vi "总磷总氮启动参数对话框.vi"() -> (2 "确认":bool, 3 "元素":cluster{"命令":string, "data":variant})   [LabVIEW 2016, in "斯坦道总磷总氮.lvlib"]
uses:
  <vilib>/Utility/miscctls.llb/LVStringsAndValuesArrayTypeDef_U16.ctl
panel:
  out "标液值":dbl caption="标液值："
  in  "取消":bool
  in  "确定":bool
  in  "测量间隔":u16
  in  "模式设置":T1(ring)
  in  "量程切换":u16(ring)=2 items=["H", "L", "AUTO"]
  in  "站号":u16(ring)=1 items=["氨氮"=3, "总磷"=1]
  in  "控制命令":T2(ring)
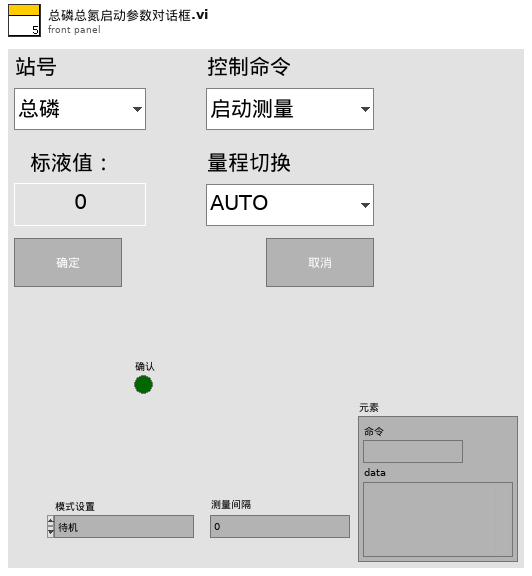
[diagram p1: front panel]
types:
  T1 = enum16{"待机", "连续模式", "周期模式", "定点模式", "受控模式", "手动模式"}
  T2 = enum16{"启动测量", "标样核查", "零点核查", "跨度核查", "空白测试", "平行样测试", "加标回收", "空白校准", "标样校准", "初始化（清洗）", "停止测试", "仪器重启", "校时", "模式设置", "测量间隔设置"}
  T3 = typedef "LVStringsAndValuesArrayTypeDef_U16.ctl" = cluster{"String":string, "Value":u16}[]
  T4 = cluster{"COD":bool, "氨氮":bool, "总氮":bool, "总磷":bool}
  T5 = cluster{"站号":u16, "量程切换":enum32{"H", "L", "AUTO"}, "控制命令":enum16{"启动测量", "标样核查", "零点核查", "跨度核查", "空白测试", "平行样测试", "加标回收", "空白校准", "标样校准", "初始化（清洗）", "停止测试", "仪器重启", "校时", "模式设置", "测量间隔设置", "盲样测试"}, "模式设置":enum16{"待机", "连续模式", "周期模式", "定点模式", "受控模式", "手动模式"}, "测量间隔":u16}
  T6 = cluster{"总磷跨度值":dbl, "总磷零点标准液浓度":dbl, "总磷跨度标准液浓度":dbl, "总磷标准液标准浓度":dbl, "总氮跨度值":dbl, "总氮零点标准液浓度":dbl, "总氮跨度标准液浓度":dbl, "总氮标准液标准浓度":dbl, "COD跨度值":dbl, "COD零点标准液浓度":dbl, "COD跨度标准液浓度":dbl, "COD标准液标准浓度":dbl, "氨氮跨度值":dbl, "氨氮零点标准液浓度":dbl, "氨氮跨度标准液浓度":dbl, "氨氮标准液标准浓度":dbl}
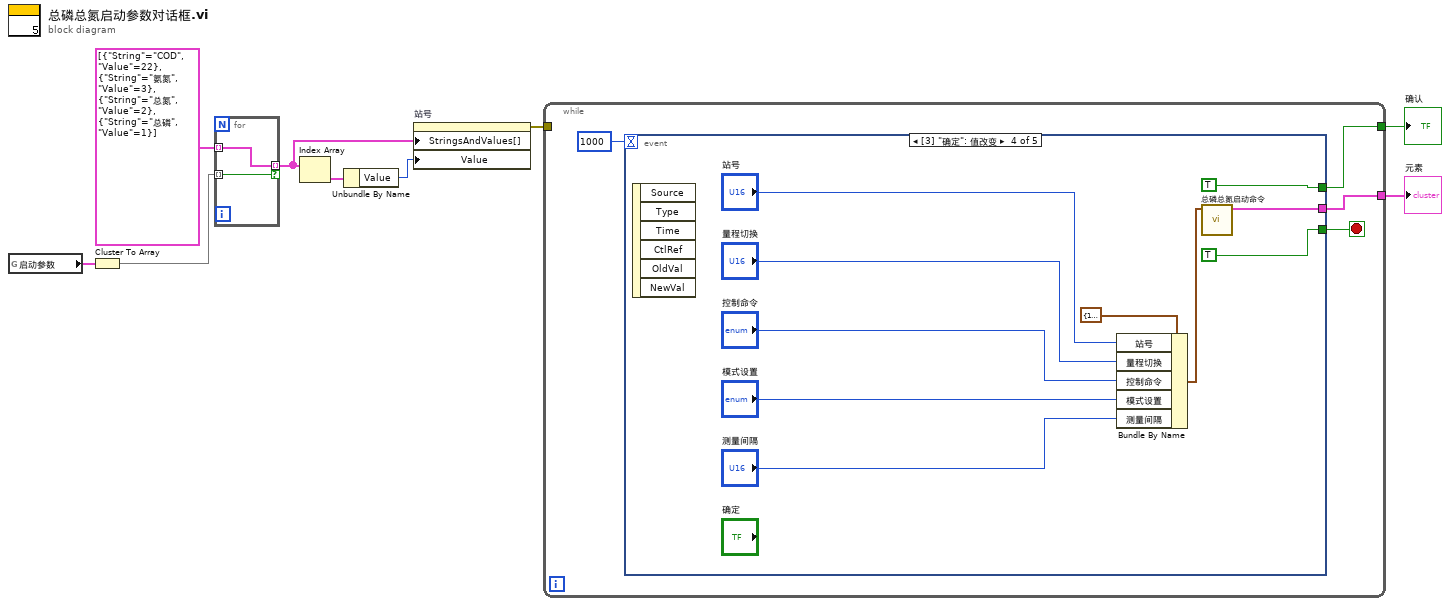
[diagram p0: block diagram]
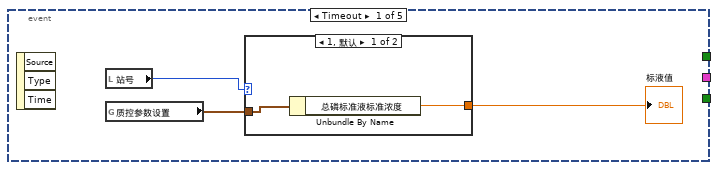
[diagram p2: hidden frame]
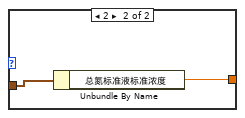
[diagram p3: hidden frame]
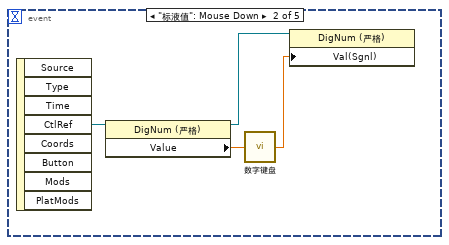
[diagram p4: hidden frame]
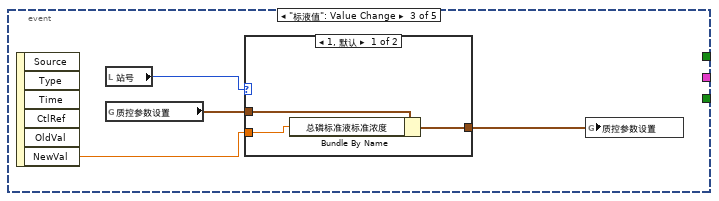
[diagram p5: hidden frame]
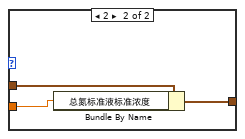
[diagram p6: hidden frame]
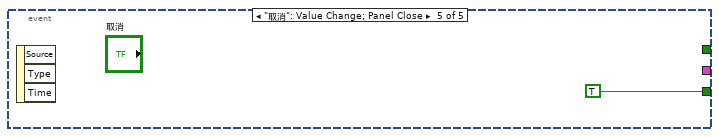
[diagram p7: hidden frame]
diagram:
  n1 = global read "总磷总氮断电保存全局变量.vi" "启动参数"() -> (w4:T4)
  n2 = Cluster To Array(cluster=w4) -> (array=w3:bool[])
  n3 = for {
    tunnel: w3 -> [w10] mode=indexing
    tunnel: T3 [{"String"="COD", "Value"=22}, {"String"="氨氮", "Value"=3}, {"String"="总氮", "Value"=2}, {"String"="总磷", "Value"=1}] ("字符串与值[]") -> [w11] mode=indexing
    tunnel: [w11] -> w1 mode=indexing if=w10
  }
  n4 = Index Array(array=w1) -> (element=w7:cluster{"String":string, "Value":u16})  [unwired: 1 in]
  n5 = Unbundle By Name(w7) -> ("Value"=w6:u16)
  n6 = property on="站号" class="Ring (严格)"("StringsAndValues[]"=w1, "Value"=w6) -> (error out=w5:errorcluster)  [unwired: 2 in, 1 out]
  n7 = while {
    tunnel: [w13] -> w9
    tunnel: [w12] -> w8
    tunnel: w5 -> [_]
    stop <- w15 stop-if-true
    n8 = event shown="[3] \"确定\": 值改变" {
      selector: _ -> [_ _ _ _ _]
      dyn-events: _ -> [_ _ _ _ _]
      timeout: 1000 -> [_ _ _ _ _]
      tunnel: [_ _ _ TRUE TRUE] -> w15
      tunnel: [_ _ _ TRUE _] -> w13
      tunnel: [_ _ _ w44 _] -> w12
      event Timeout {
        n9 = event-data() -> ()  [unwired: 1 in, 3 out]
        n10 = local read "站号"() -> (w17:u16)
        n11 = global read "总磷总氮断电保存全局变量.vi" "质控参数设置"() -> (w18:T6)
        n12 = case shown="1, 默认" w17 {
          tunnel: w18 -> [w20 w22]
          tunnel: [w19 w21] -> w16
          frame 1, Default {
            n13 = Unbundle By Name(w20) -> ("总磷标准液标准浓度"=w19:dbl)
          }
          frame 2 {
            n14 = Unbundle By Name(w22) -> ("总氮标准液标准浓度"=w21:dbl)
          }
        }
        "标液值" <- w16
      }
      event "标液值": Mouse Down {
        n15 = event-data() -> ("CtlRef"=w26:refnum<vi>)  [unwired: 1 in, 7 out]
        n16 = property class="DigNum (严格)"(reference=w26) -> (reference out=w23:refnum<vi>, "Value"=w25:dbl)  [unwired: 1 in, 1 out]
        n17 = call "数字键盘.vi"("OldNumber"=w25) -> ("NewNumber"=w24:dbl)
        n18 = property class="DigNum (严格)"(reference=w23, "Val(Sgnl)"=w24) -> ()  [unwired: 1 in, 2 out]
      }
      event "标液值": Value Change {
        n19 = event-data() -> ("NewVal"=w28:dbl)  [unwired: 1 in, 5 out]
        n20 = local read "站号"() -> (w30:u16)
        n21 = global read "总磷总氮断电保存全局变量.vi" "质控参数设置"() -> (w29:T6)
        n22 = case shown="1, 默认" w30 {
          tunnel: w29 -> [w33 w36]
          tunnel: [w31 w34] -> w27
          tunnel: w28 -> [w32 w35]
          frame 1, Default {
            n23 = Bundle By Name(cluster=w33, "总磷标准液标准浓度"=w32) -> (w31:T6)
          }
          frame 2 {
            n24 = Bundle By Name(cluster=w36, "总氮标准液标准浓度"=w35) -> (w34:T6)
          }
        }
        n25 = global write "总磷总氮断电保存全局变量.vi" "质控参数设置"(w27) -> ()
      }
      event "确定": Value Change {
        n26 = event-data() -> ()  [unwired: 1 in, 6 out]
        n27 = Bundle By Name(cluster=T5 {"站号"=1, "量程切换"=enum."AUTO", "控制命令"=enum."启动测量", "模式设置"=enum."待机", "测量间隔"=0} ("参数"), "站号"="站号", "量程切换"="量程切换", "控制命令"="控制命令", "模式设置"="模式设置", "测量间隔"="测量间隔") -> (w42:T5)
        n28 = call "总磷总氮启动命令.vi"("参数"=w42) -> ("启动命令"=w44:cluster{"命令":string, "data":variant})  [unwired: 10 in]
      }
      event "取消": Value Change; Panel Close {
        n29 = event-data() -> ()  [unwired: 1 in, 3 out]
      }
    }
  }
  "元素" <- w8
  "确认" <- w9
